vi "DQMH-GenNet Get Notifier From Variant.vi"(10 "error in":errorcluster, 11 "Message Data Variant":variant) -> (2 "error out":errorcluster, 3 "Wait Notifier":refnum<notifier>)   [LabVIEW 2014, in "hse-gennet.lvlib"]
doc: "HSE: Gets the Wait Notifier Refnum (datatype variant) from the Message Data variant\n\n____\nHAMPEL SOFTWARE ENGINEERING v0.7.0 (2018-07-16 18:12)"
uses:
  hse-gennet.lvlib
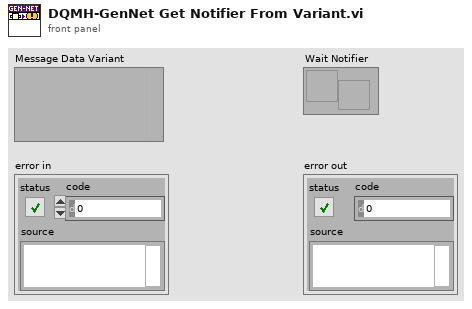
[diagram p1: front panel]
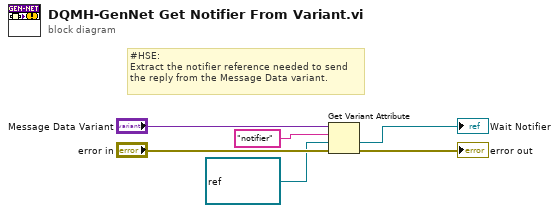
[diagram p0: block diagram]
diagram:
  # "#HSE: \nExtract the notifier reference needed to send\nthe reply from the Message Data variant."
  n1 = Get Variant Attribute(Variant="Message Data Variant", name="notifier", default value (empty Variant)=refnum<notifier> refnum ("Wait Notifier"), error in="error in") -> (value=→"Wait Notifier":refnum<notifier>, error out=→"error out":errorcluster)  [unwired: 2 out]
